vi "Calc DC RMS Peak Freq.vi"(0 "input data":fxp<+/-,16,16>, 1 "reset":bool, 5 "Sample Size (1k)":u16=1000) -> (4 "DC":fxp<+/-,16,16>, 6 "RMS":fxp<+,16,16>, 8 "Peak":fxp<+/-,16,16>, 10 "Frequency (Hz)":sgl, 14 "output valid":bool)   [LabVIEW 2014]
doc: "Calculates the DC (mean) and/or RMS values of an input signal. You also can use this VI to calculate the intermediate sum, mean square, or square sum values in order to save FPGA resources.\n--------------------\n\nThis Express VI is configured as follows:\n\n<b>Measurement Time Setup</b>\nNumber of samples: 1000\nMeasurement time: 20ms\nSample rate: 50kS/s\n\n<b>Windowing</b>\nNone\n\n<b>Measurements</b>\nDC (Mean)\nRMS\n\n<b>Execution Mode</b>\nOutside single-cycle Timed Loop"
uses:
  <vilib>/Platform/TimedLoop/XDataNode/timing_clust.ctl
  <vilib>/Platform/TimedLoop/XDataNode/nitl_modes.ctl
  <vilib>/Platform/TimedLoop/XDataNode/wakeup.ctl
  <vilib>/rvi/FXPMathLib/basic elements/FxpIntAccumulator/subVIs/nifxpmath_IntAccumulator_SimConfig.ctl
  <vilib>/rvi/FXPMathLib/FxpSqrt/subVIs/nifxpmath_Sqrt_SimConfig.ctl
  <vilib>/fxp/LVFixedPointOverflowPolicyTypeDef.ctl
  <vilib>/rvi/FXPMathLib/basic elements/FxpIntAccumulator/simVIs/DllFxpIntAccumulator_sub.vi
  <vilib>/rvi/FXPMathLib/FxpSqrt/simVIs/DllSqrtTemp_sub.vi
  <vilib>/rvi/Analysis/utilities/niFPGA Threshold Crossing Logic.vi
  <vilib>/Platform/TimedLoop/XDataNode/XDataNode.xnode
  <vilib>/rvi/Analysis/measure/period/templates/niFPGA Period Edge Direction.ctl
  <vilib>/rvi/FXPMathLib/basic elements/FxpIntAccumulator/XNode/nifxpmath_IntAccumulator.xnode
  <vilib>/rvi/FXPMathLib/FxpMul/XNode/nifxpmath_Multiplier.xnode
  <vilib>/rvi/FXPMathLib/FxpSqrt/XNode/nifxpmath_Sqrt.xnode
  <vilib>/rvi/Analysis/measure/period/XNode/niFpgaAnalogPeriod.xnode
  <vilib>/Platform/TimedLoop/XDataNode/XDNodeRunTimeDep.lvlib
  <vilib>/rvi/FXPMathLib/sim/FxpSim.dll
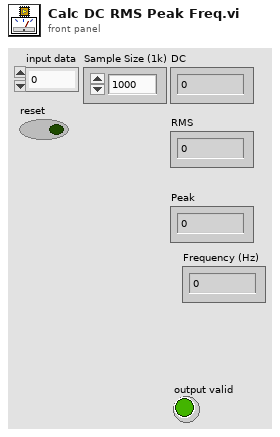
[diagram p1: front panel]
types:
  T1 = typedef "XDNodeRunTimeDep.lvlib/timing_clust.ctl" = cluster{"Expected End [f-1]":u64, "Actual End [f-1]":u64, "Finished Late? [f-1]":bool, "Expected End [i-1]":u64, "Actual End [i-1]":u64, "Finished Late? [i-1]":bool, "Expected Start [i]":u64, "Actual Start [i]":u64, "Expected Start [f]":u64, "Actual Start [f]":u64, "Source Name":string, "Structure Name":string, "Period":i64, "Deadline":i64, "Offset":i64, "Start":i64, "Priority":i32, "Timeout":i32, "Mode":T2, "Wakeup Reason":T3, "Error":errorcluster, "Source Type":string, "Secondary Source Type":string, "Global End Time":u64, "Global Start Time":u64, "Frame Duration":u64, "Iteration Duration":u64, "Assigned CPU":i32, "I/O Scan Engine Mode":u32}
  T2 = typedef "XDNodeRunTimeDep.lvlib/nitl_modes.ctl" = enum32{"No Change", "Process missed periods, maintain original phase", "Discard missed periods, maintain original phase", "Process missed periods, ignore original phase", "Discard missed periods, ignore original phase"}
  T3 = typedef "XDNodeRunTimeDep.lvlib/wakeup.ctl" = enum32{"Normal", "Aborted", "Asynchronous wakeup", "Timing source error", "Timed loop error", "Timeout"}
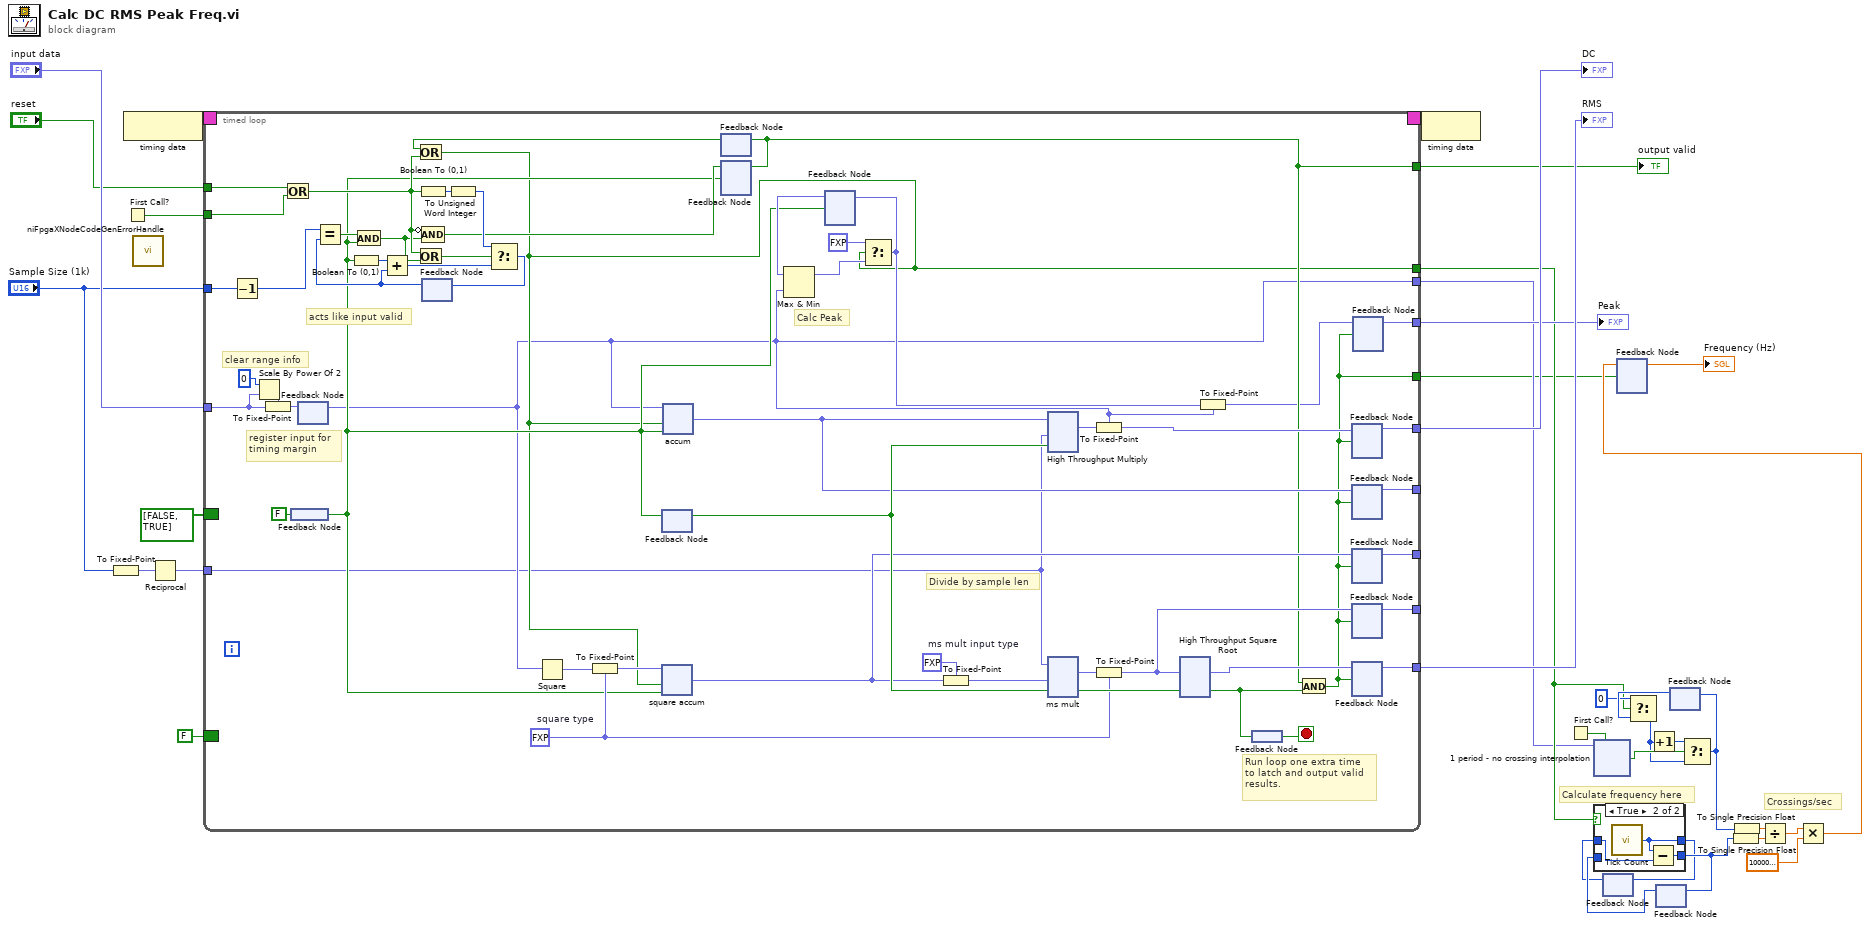
[diagram p0: block diagram]
diagram:
  # "Crossings/sec"
  # "Calculate frequency here"
  n1 = To Fixed-Point(number="Sample Size (1k)") -> (fixed-point=w3:fxp<+,16,16>)  [unwired: 1 in]
  n2 = First Call?() -> (First Call?: T/F=w25:bool)
  n3 = node-c288() -> (w29:T1)
  n4 = call <vilib>:"niFpgaXNodeCodeGenErrorHandle.vi"() -> ()  [unwired: 1 in]
  n5 = Reciprocal(x=w3) -> (1/x=w1:fxp<+,17,1>)
  n6 = timed-loop {
    tunnel: "input data" -> [w56]
    tunnel: "reset" -> [w85]
    tunnel: w25 -> [w84]
    tunnel: [w42] -> w30
    timing: w29 -> [_]
    timing-out: [_] -> w28
    border: bool[] [FALSE, TRUE] -> [_]
    tunnel: [w63] -> _
    tunnel: [w62] -> _
    tunnel: [w61] -> _
    tunnel: [w60] -> w32
    tunnel: [w65] -> w31
    border: FALSE ("output valid") -> [_]
    tunnel: "Sample Size (1k)" -> [w47]
    tunnel: [w43] -> w24
    tunnel: [w38] -> w8
    tunnel: [w37] -> w7
    tunnel: [w36] -> w4
    tunnel: w1 -> [w35]
    stop <- w64 stop-if-true
    w49 = fxp<+,34,40> 0.0  # ms mult input type
    w74 = fxp<+,31,31> 0.0  # square type
    # "Divide by sample len"
    # "Calc Peak"
    # "register input for \ntiming margin"
    # "Run loop one extra time\nto latch and output valid\nresults."
    # "clear range info"
    # "acts like input valid"
    n7 = Decrement(x=w47) -> (x-1=w48:u16)
    n8 = Scale By Power Of 2(n=0, x=w56) -> (x*2^n=w59:fxp<+/-,16,16>)
    n9 = To Fixed-Point(fixed-point type=w59, number=w56) -> (fixed-point=w57:fxp<+/-,16,16>)
    n10 = Or(x=w85, y=w84) -> (x .or. y?=w79:bool)
    n11 = feedback #1() -> (w41:bool)
    n12 = feedback-in #1(FALSE) -> ()
    n13 = feedback-in #2(w57) -> ()
    n14 = feedback #2() -> (w37:fxp<+/-,16,16>)  [unwired: 1 in]
    n15 = Boolean To (0,1)(Boolean=w41) -> (0, 1=w83:i16)
    n16 = Boolean To (0,1)(Boolean=w79) -> (0, 1=w88:i16)
    n17 = feedback #3() -> (w76:u16)  [unwired: 1 in]
    n18 = Equal?(x=w48, y=w76) -> (x = y?=w81:bool)
    n19 = And(x=w81, y=w41) -> (x .and. y?=w78:bool)
    n20 = Add(x=w83, y=w76) -> (x+y=w82:u16)
    n21 = Or(x=w79, y=w78) -> (x .or. y?=w80:bool)
    n22 = Compound Arithmetic op=AND(invert w79, w78) -> (w73:bool)
    n23 = To Unsigned Word Integer(number=w88) -> (unsigned 16bit integer=w87:u16)
    n24 = Select(t=w87, s=w80, f=w82) -> (s? t:f=w86:u16)
    n25 = feedback-in #3(w86) -> ()
    n26 = Square(x=w37) -> (x^2=w53:fxp<+,31,31>)
    n27 = To Fixed-Point(fixed-point type=w74, number=w53) -> (fixed-point=w52:fxp<+,31,31>)
    n28 = feedback-in #4(w41) -> ()
    n29 = feedback #4() -> (w72:bool)  [unwired: 1 in]
    n30 = feedback #5() -> (w77:bool)  [unwired: 1 in]
    n31 = Or(x=w77, y=w79) -> (x .or. y?=w38:bool)
    n32 = xnode "square accum"("x"=w52, "load (F)"=w38, "enable (T)"=w41) -> ("s"=w70:fxp<+,40,40>)  [unwired: 2 in, 1 out]
    n33 = xnode "accum"("x"=w37, "load (F)"=w38, "enable (T)"=w41) -> ("s"=w69:fxp<+/-,26,26>)  [unwired: 2 in, 1 out]
    n34 = feedback-in #6(w73, w41) -> ()
    n35 = feedback #6() -> (w42:bool)  [unwired: 1 in]
    n36 = feedback-in #5(w42) -> ()
    n37 = feedback #7() -> (w45:fxp<+/-,32,20>)  [unwired: 1 in]
    n38 = Max & Min(x=w45, y=w37) -> (max(x,y)=w44:fxp<+/-,32,20>)  [unwired: 1 out]
    n39 = Select(t=fxp<+/-,32,20> 0.0, s=w38, f=w44) -> (s? t:f=w40:fxp<+/-,32,20>)
    n40 = feedback-in #7(w40, w41) -> ()
    n41 = To Fixed-Point(fixed-point type=w49, number=w70) -> (fixed-point=w50:fxp<+,34,40>)
    n42 = xnode ("High Throughput Multiply")("x"=w69, "y"=w35, "input valid"=w72) -> ("x*y"=w54:fxp<+/-,43,27>)  [unwired: 1 in, 2 out]
    n43 = xnode ("ms mult")("x"=w35, "y"=w50, "input valid"=w72) -> ("x*y"=w51:fxp<+,51,41>, "output valid"=w75:bool)  [unwired: 1 in, 1 out]
    n44 = To Fixed-Point(fixed-point type=w37, number=w54) -> (fixed-point=w68:fxp<+/-,16,16>)
    n45 = To Fixed-Point(fixed-point type=w74, number=w51) -> (fixed-point=w67:fxp<+,31,31>)
    n46 = xnode ("High Throughput Square Root")("x"=w67, "input valid"=w75) -> ("sqrt(x)"=w66:fxp<+,16,16>, "output valid"=w55:bool)  [unwired: 1 in, 1 out]
    n47 = To Fixed-Point(fixed-point type=w37, number=w40) -> (fixed-point=w39:fxp<+/-,16,16>)
    n48 = feedback-in #8(w55) -> ()
    n49 = feedback #8() -> (w64:bool)
    n50 = And(x=w42, y=w55) -> (x .and. y?=w36:bool)
    n51 = feedback #9() -> (w60:fxp<+/-,16,16>)  [unwired: 1 in]
    n52 = feedback-in #9(w68, w36) -> ()
    n53 = feedback #10() -> (w61:fxp<+/-,26,26>)  [unwired: 1 in]
    n54 = feedback-in #10(w69, w36) -> ()
    n55 = feedback #11() -> (w62:fxp<+,40,40>)  [unwired: 1 in]
    n56 = feedback-in #11(w70, w36) -> ()
    n57 = feedback #12() -> (w63:fxp<+,31,31>)  [unwired: 1 in]
    n58 = feedback-in #12(w67, w36) -> ()
    n59 = feedback #13() -> (w65:fxp<+,16,16>)  [unwired: 1 in]
    n60 = feedback-in #13(w66, w36) -> ()
    n61 = feedback #14() -> (w43:fxp<+/-,16,16>)  [unwired: 1 in]
    n62 = feedback-in #14(w39, w36) -> ()
  }
  "DC" <- w32
  "RMS" <- w31
  "output valid" <- w30
  "Peak" <- w24
  n63 = node-c288(w28) -> ()
  n64 = First Call?() -> (First Call?: T/F=w22:bool)
  n65 = xnode ("1 period - no crossing interpolation")("input data"=w7, "reset"=w22) -> ("crossing"=w23:bool)  [unwired: 3 in, 3 out]
  n66 = feedback #15() -> (w14:u32)  [unwired: 1 in]
  n67 = feedback #16() -> (→"Frequency (Hz)":sgl)  [unwired: 1 in]
  n68 = feedback #17() -> (w15:u32)  [unwired: 1 in]
  n69 = case shown="True" w8 {
    tunnel: [w170 w173] -> w13
    tunnel: w14 -> [w170 w172]
    tunnel: [w169 w171] -> w16
    tunnel: w15 -> [w169 _]
    frame False {
    }
    frame True {
      n70 = call "Tick Count"() -> ("Tick Count(uSec)"=w173:u32)
      n71 = Subtract(x=w173, y=w172) -> (x-y=w171:u32)
    }
  }
  n72 = feedback-in #15(w13) -> ()
  n73 = feedback-in #17(w16) -> ()
  n74 = feedback #18() -> (w12:u16)  [unwired: 1 in]
  n75 = Select(t=u16 0, s=w8, f=w12) -> (s? t:f=w11:u16)
  n76 = Increment(x=w11) -> (x+1=w9:u16)
  n77 = Select(t=w9, s=w23, f=w11) -> (s? t:f=w19:u16)
  n78 = feedback-in #18(w19) -> ()
  n79 = To Single Precision Float(number=w16) -> (single precision float=w18:sgl)
  n80 = To Single Precision Float(number=w19) -> (single precision float=w17:sgl)
  n81 = Divide(x=w17, y=w18) -> (x/y=w20:sgl)
  n82 = Multiply(x=w20, y=sgl 1000000.0) -> (x*y=w6:sgl)
  n83 = feedback-in #16(w6, w4) -> ()
